vi "libssh2_session_init_ex.vi"(7 "abstract":T1, 8 "error in (no error)":errorcluster, 9 "myrealloc (0 = NULL)":u64, 10 "myfree (0 = NULL)":u64, 11 "myalloc (0 = NULL)":u64) -> (0 "error out":errorcluster, 3 "session":T2)   [LabVIEW 2017, in "libssh2.lvlib"]
doc: "Initialize a session with abstract data.\n\nThis function utilizes the lvssh2 extension library to register <B>abstract</B> function callbacks. You can disable the extension library by defining the LVSSH2_NO_EXTENSIONS conditional disable symbol with the value 'True' in the project properties. When the extension library is disabled, the <B>abstract</B> function callbacks are not registered."
uses:
  libssh2.lvlib
  Session Refnum.ctl
  libssh2_session_abstract.ctl
  Global Settings.vi
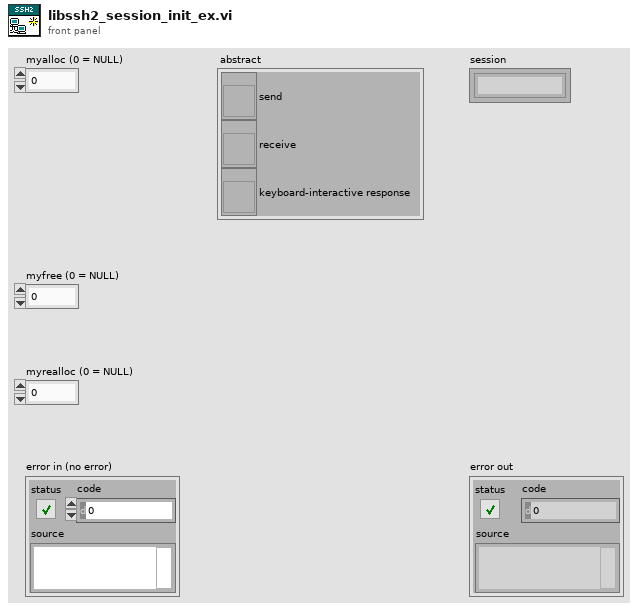
[diagram p1: front panel]
types:
  T1 = typedef "libssh2.lvlib/libssh2_session_abstract.ctl" = cluster{"send":refnum<vi>, "receive":refnum<vi>, "keyboard-interactive response":refnum<vi>}
  T2 = typedef "libssh2.lvlib/Session Refnum.ctl" = refnum<k1>
  T3 = typedef "libssh2.lvlib/lvssh2_session_callback_events.ctl" = cluster{"32-bit":cluster{"send":refnum<user-event>, "recv":refnum<user-event>, "kbdint_response":refnum<user-event>}, "64-bit":cluster{"send":refnum<user-event>, "recv":refnum<user-event>, "kbdint_response":refnum<user-event>}, "stop":cluster{"send":refnum<user-event>, "recv":refnum<user-event>, "kbdint_response":refnum<user-event>}}
  T4 = cluster{"send":refnum<user-event>, "recv":refnum<user-event>, "kbdint_response":refnum<user-event>}
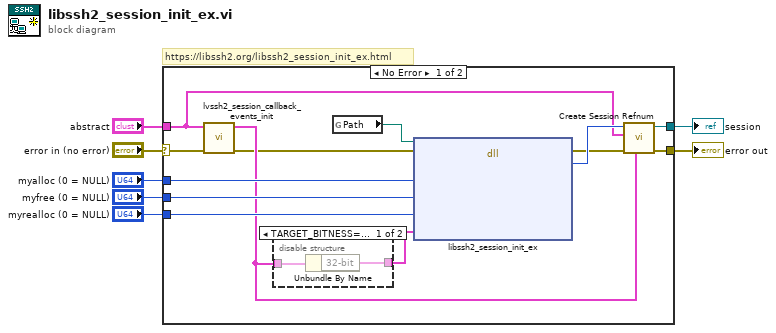
[diagram p0: block diagram]
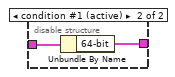
[diagram p2: hidden frame]
diagram:
  # "https://libssh2.org/libssh2_session_init_ex.html"
  n1 = case shown="No Error" "error in (no error)" {
    selector: "error in (no error)" -> [w12 w25]
    tunnel: "myalloc (0 = NULL)" -> [w20 _]
    tunnel: "myfree (0 = NULL)" -> [w19 _]
    tunnel: "myrealloc (0 = NULL)" -> [w18 _]
    tunnel: [w16 _] -> w4
    tunnel: [w14 w25] -> w3
    tunnel: "abstract" -> [w11 _]
    frame No Error {
      n2 = call "lvssh2_session_callback_events_init.vi"("error in (no error)"=w12, "abstract"=w11) -> ("error out"=w8:errorcluster, "events"=w10:T3)  [unwired: 8 in]
      n3 = disable-structure shown="TARGET_BITNESS==32, Default" {
        disable-tunnel: w10 -> [w22 w24]
        disable-tunnel: [w21 w23] -> w9
        frame condition #0 {
          n4 = Unbundle By Name(w22) -> ("32-bit"=w21:T4)
        }
        frame condition #1 (active) {
          n5 = Unbundle By Name(w24) -> ("64-bit"=w23:T4)
        }
      }
      n6 = global read "Global Settings.vi" "Path"() -> (w13:path)
      n7 = dll-call lib="?" fn="libssh2_session_init_ex"(path in=w13, error in=w8, "myalloc"=w20, "myfree"=w19, "myrealloc"=w18, "events"=w9) -> (error out=w15:errorcluster, "return value"=w17:u64)  [unwired: 5 in, 1 out]
      n8 = call "Create Session Refnum.vi"("events"=w10, "error in (no error)"=w15, "abstract"=w11, "LIBSSH2_SESSION*"=w17) -> ("error out"=w14:errorcluster, "session"=w16:T2)  [unwired: 6 in]
    }
    frame Error {
    }
  }
  "session" <- w4
  "error out" <- w3
